vi "Process Packet.vi"(8 "error in (no error)":errorcluster, 10 "ServerRequest":refnum<class "ControlPacket.lvclass">, 11 "Session.Server":refnum<class "Session.Server.lvclass">) -> (0 "error out":errorcluster, 3 "Session.Server":refnum<class "Session.Server.lvclass">)   [LabVIEW 2013, in "MQTT Server.lvlib" / "Session.Server.lvclass"]
uses:
  Session.Server.lvclass
  <vilib>/LabVIEW Open Source Project/MQTT Control Packets/Control Packets/ControlPacket/ControlPacket.lvclass
  MQTT_Base/Session/Session.lvclass
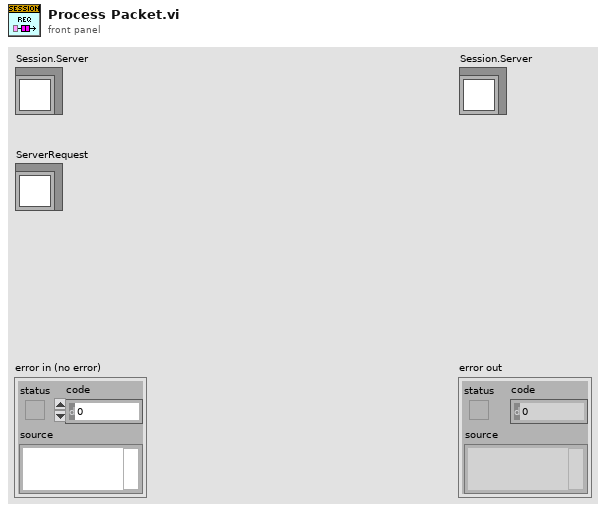
[diagram p1: front panel]
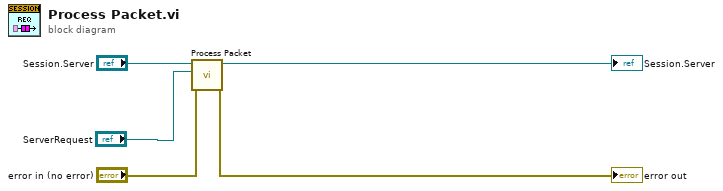
[diagram p0: block diagram]
diagram:
  n1 = call-parent "Process Packet.vi"("error in (no error)"="error in (no error)", "Incoming Packet"="ServerRequest", "Session in"="Session.Server") -> ("error out"=→"error out":errorcluster, "Session out"=→"Session.Server":refnum<class "Session.Server.lvclass">)  [unwired: 7 in]
